vi "Create new file.vi"(0 "reference in":refnum<class "TDMS_DataHandler.lvclass">, 5 "error in (no error)":errorcluster) -> (14 "reference out":refnum<class "TDMS_DataHandler.lvclass">, 15 "TDMS ref out-":refnum<k34>, 19 "error out":errorcluster)   [LabVIEW 2019, in "TDMS_DataHandler.lvclass"]
doc: "Creates a new blank tdms file for manipulation"
uses:
  TDMS_DataHandler.lvclass
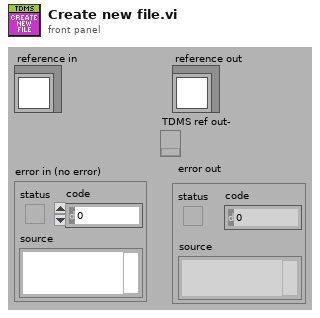
[diagram p1: front panel]
types:
  T1 = enum16{"open", "open or create", "create or replace", "create", "open (read-only)"}
  T2 = typedef "TDMS_DataHandler.lvclass/ObjectAttributesRef.ctl" = refnum<data-value>
  T3 = typedef "TDMS_DataHandler.lvclass/ObjectAttributes.ctl" = cluster{"Directory":path, "FilePath":path, "FileRef":refnum<k34>, "ExperimentName":string, "GroupName":string, "ChannelNames":string[], "Datum":waveform(dbl)[], "Group_Metadata":cluster{"property names":string[], "property values":variant[]}, "Channel_Metadata":cluster{"property names":string[], "property values":variant[]}}
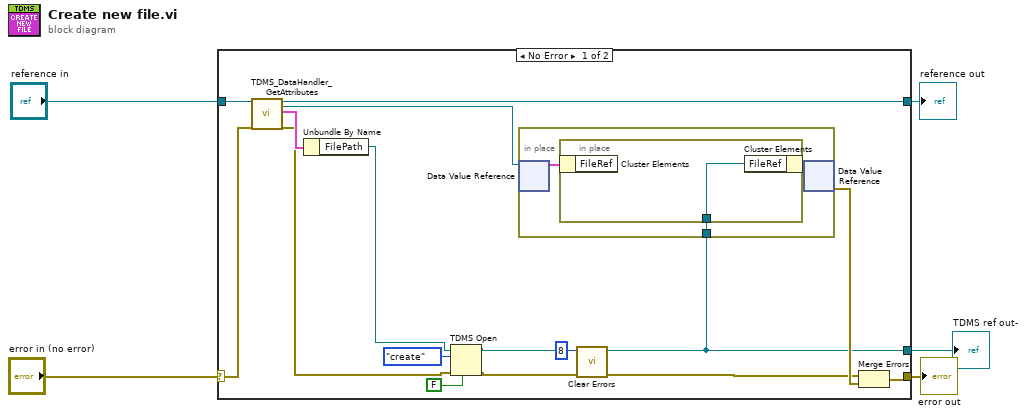
[diagram p0: block diagram]
diagram:
  n1 = case shown="No Error" "error in (no error)" {
    selector: "error in (no error)" -> [w18 w26]
    tunnel: [w15 w26] -> w4
    tunnel: [w19 w25] -> w2
    tunnel: "reference in" -> [w20 w25]
    tunnel: [w9 _] -> w1
    frame No Error {
      n2 = call "TDMS_DataHandler_GetAttributes.vi"("reference in"=w20, "error in (no error)"=w18) -> ("reference out"=w19:refnum<class "TDMS_DataHandler.lvclass">, "attributes ref"=w16:T2, "attributes"=w14:T3, "error out"=w11:errorcluster)  [unwired: 14 in]
      n3 = Unbundle By Name(w14) -> ("FilePath"=w6:path)
      n4 = TDMS Open(6:FALSE ("disable buffering? (T)"), 8:w11, 10:T1."create" ("operation (0:open)"), 11:w6) -> (0:w10:errorcluster, 3:w9:refnum<k34>)  [unwired: 3 in]
      n5 = in-place {
        in-place-border: w9 -> [w21]
        n6 = in-place-dvr #1(w16) -> (w22:T3)  [unwired: 1 out]
        n7 = in-place {
          in-place-border: w21 -> [w24]
          n8 = in-place-cluster #2(w22) -> ()  [unwired: 1 out]
          n9 = in-place-cluster #2("FileRef"=w24) -> (w23:T3)
        }
        n10 = in-place-dvr #1(w23) -> (w17:errorcluster)  [unwired: 1 out]
      }
      n11 = call <vilib>:"Clear Errors.vi"("error in (no error)"=w10, "specific error code to clear (0: all)"=8) -> ("error out"=w13:errorcluster)  [unwired: 4 in, 1 out]
      n12 = Merge Errors(w13, w17) -> (w15:errorcluster)
    }
    frame Error {
    }
  }
  "error out" <- w4
  "reference out" <- w2
  "TDMS ref out-" <- w1
